vi "SendMessageInternal.vi"(6 "timeout (5 sec)":i32=5000, 8 "error in (no error)":errorcluster, 10 "message":T1, 11 "connection ID in":T4) -> (0 "error out":errorcluster, 3 "connection ID out":T4)   [LabVIEW 2017, in "ServerComm.lvlib"]
uses:
  <vilib>/addons/InsightCM/Devices/Shared/Common/ServerComm/ServerComm.lvlib
  <vilib>/addons/InsightCM/MessageBus/TcpApi/controls/TcpMessageReference.ctl
  <vilib>/addons/InsightCM/MessageBus/Base/controls/Message.ctl
  <vilib>/addons/InsightCM/MessageBus/Base/controls/MessageHeader.ctl
  <vilib>/addons/InsightCM/MessageBus/Base/controls/KeyValuePair.ctl
  <vilib>/addons/InsightCM/Utilities/PropertyHelpers/PropertyHelpers.lvlib
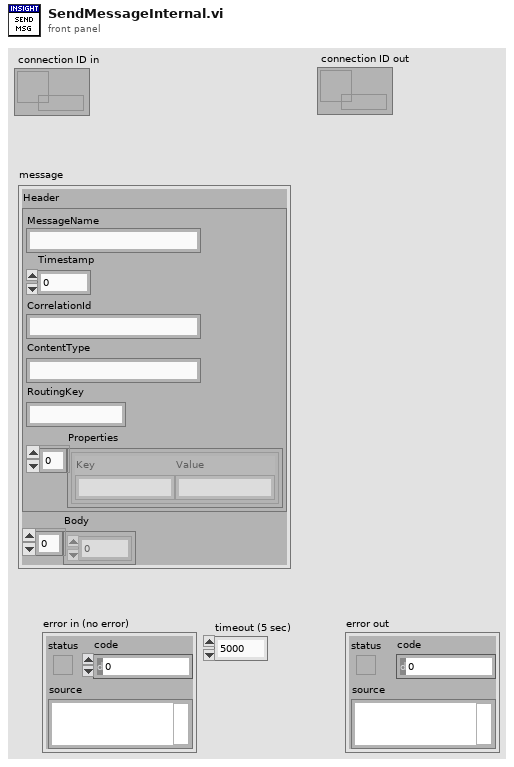
[diagram p1: front panel]
types:
  T1 = typedef "Message.ctl" = cluster{"Header":T2, "Body":u8[]}
  T2 = typedef "MessageHeader.ctl" = cluster{"MessageName":string, "Timestamp":i64, "CorrelationId":string, "ContentType":string, "RoutingKey":string, "Properties":T3[]}
  T3 = typedef "KeyValuePair.ctl" = cluster{"Key":string, "Value":string}
  T4 = typedef "TcpMessageReference.ctl" = refnum<data-value>
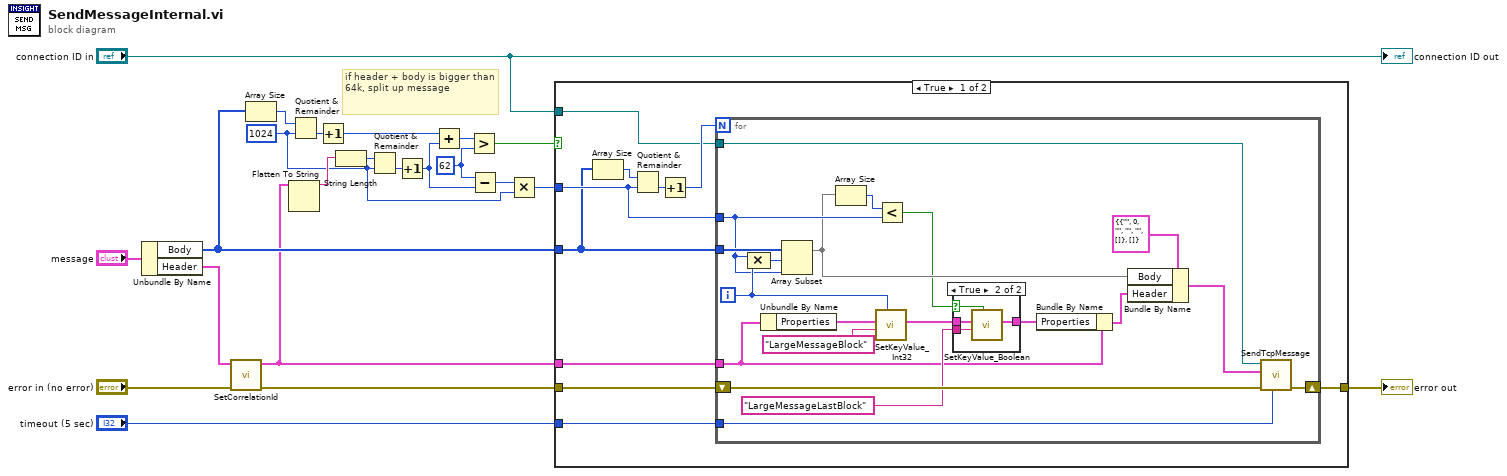
[diagram p0: block diagram]
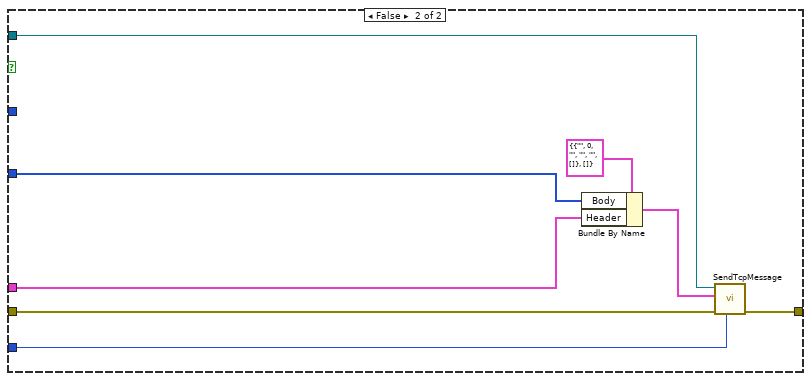
[diagram p3: hidden frame]
diagram:
  w13 = 62 ("y")
  w1 = 1024 ("y")
  # "if header + body is bigger than 64k, split up message"
  n1 = Unbundle By Name("message") -> ("Body"=w9:u8[], "Header"=w21:T2)
  n2 = call <vilib>:"SetCorrelationId.vi"("error in (no error)"="error in (no error)", "header in"=w21) -> ("error out"=w6:errorcluster, "header out"=w8:T2)  [unwired: 7 in, 1 out]
  n3 = Array Size(array=w9) -> (size(s)=w16:i32)
  n4 = Flatten To String(anything=w8) -> (data string=w20:string)  [unwired: 3 in, 2 out]
  n5 = Quotient & Remainder(x=w16, y=w1) -> (floor(x/y)=w17:i32)  [unwired: 1 out]
  n6 = Increment(x=w17) -> (x+1=w14:i32)
  n7 = String Length(string=w20) -> (length=w18:i32)
  n8 = Quotient & Remainder(x=w18, y=w1) -> (floor(x/y)=w19:i32)  [unwired: 1 out]
  n9 = Increment(x=w19) -> (x+1=w12:i32)
  n10 = Add(x=w14, y=w12) -> (x+y=w15:i32)
  n11 = Greater?(x=w15, y=w13) -> (0:w4:bool)
  n12 = Subtract(x=w13, y=w12) -> (x-y=w3:i32)
  n13 = Multiply(x=w3, y=w1) -> (x*y=w2:i32)
  n14 = case shown="True" w4 {
    tunnel: w2 -> [w29 _]
    tunnel: [w28 w65] -> w10
    tunnel: w9 -> [w27 w58]
    tunnel: w8 -> [w26 w59]
    tunnel: "connection ID in" -> [w25 w64]
    tunnel: w6 -> [w24 w63]
    tunnel: "timeout (5 sec)" -> [w23 w62]
    frame True {
      n15 = Array Size(array=w27) -> (size(s)=w32:i32)
      n16 = Quotient & Remainder(x=w32, y=w29) -> (floor(x/y)=w30:i32)  [unwired: 1 out]
      n17 = Increment(x=w30) -> (x+1=w31:i32)
      n18 = for {
        N: w31 -> [_]
        tunnel: w27 -> [w52]
        shift-right: [w49] -> w28
        shift-left: w24 -> [w50]
        tunnel: w29 -> [w42]
        tunnel: w26 -> [w41]
        tunnel: w25 -> [w37]
        tunnel: w23 -> [w33]
        i -> [w47]
        n19 = Compound Arithmetic op=MULTIPLY(w42, w47) -> (w51:i32)
        n20 = Unbundle By Name(w41) -> ("Properties"=w46:T3[])
        n21 = Array Subset(array=w52, index=w51, length=w42) -> (w38:u8[])
        n22 = Array Size(array=w38) -> (size(s)=w43:i32)
        n23 = call <vilib>:"SetKeyValue_Int32.vi"("value"=w47, "key"="LargeMessageBlock", "key value pairs"=w46) -> ("key value pairs out"=w45:T3[])  [unwired: 8 in]
        n24 = Less?(x=w43, y=w42) -> (x < y?=w34:bool)
        n25 = case shown="True" w34 {
          selector: w34 -> [_ w54]
          tunnel: w45 -> [w53 w57]
          tunnel: "LargeMessageLastBlock" ("key") -> [_ w56]
          tunnel: [w53 w55] -> w40
          frame False {
          }
          frame True {
            n26 = call <vilib>:"SetKeyValue_Boolean.vi"("value"=w54, "key"=w56, "key value pairs"=w57) -> ("key value pairs out"=w55:T3[])  [unwired: 8 in]
          }
        }
        n27 = Bundle By Name(cluster=w41, "Properties"=w40) -> (w35:T2)
        n28 = Bundle By Name(cluster=T1 {"Header"={"MessageName"="", "Timestamp"=0, "CorrelationId"="", "ContentType"="", "RoutingKey"="", "Properties"=[]}, "Body"=[]} ("message"), "Body"=w38, "Header"=w35) -> (w36:T1)
        n29 = call <vilib>:"SendTcpMessage.vi"("timeout (5 sec)"=w33, "error in (no error)"=w50, "message"=w36, "connection ID in"=w37) -> ("error out"=w49:errorcluster)  [unwired: 5 in, 2 out]
      }
    }
    frame False {
      n30 = Bundle By Name(cluster=T1 {"Header"={"MessageName"="", "Timestamp"=0, "CorrelationId"="", "ContentType"="", "RoutingKey"="", "Properties"=[]}, "Body"=[]} ("message"), "Body"=w58, "Header"=w59) -> (w60:T1)
      n31 = call <vilib>:"SendTcpMessage.vi"("timeout (5 sec)"=w62, "error in (no error)"=w63, "message"=w60, "connection ID in"=w64) -> ("error out"=w65:errorcluster)  [unwired: 5 in, 2 out]
    }
  }
  "error out" <- w10
  "connection ID out" <- "connection ID in"
